vi "Detected DPIs.vi"() -> (0 "error out":errorcluster, 2 "DPI resources":string[](array[string]))   [LabVIEW 2021, in "Audio ADC Shared.lvlib"]
uses:
  Audio ADC Shared.lvlib
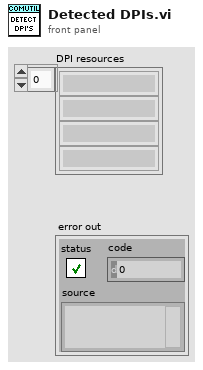
[diagram p1: front panel]
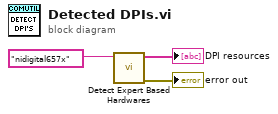
[diagram p0: block diagram]
diagram:
  n1 = call "Detect Expert Based Hardwares.vi"("Expert name"="nidigital657x") -> ("error out"=→"error out":errorcluster, "Alias names"=→"DPI resources":string[])  [unwired: 8 in, 1 out]
